vi "Window-Stage modulation program.vi"() -> ()   [LabVIEW 2020]
uses:
  Peripherals Control/XYZ Stage/Pos Modulator VIs/Typedefs/Motion Mode.ctl
  Peripherals Control/XYZ Stage/Pos Modulator VIs/Typedefs/Ops.ctl
  <vilib>/GPower/Comparison/Library/IsEven/IsEvenI32.vi
  <vilib>/GPower/Comparison/GPComparison.lvlib
panel:
  in  "Speed (um/sec)":dbl=30000.0
  in  "Z Step Size (um)":dbl=5.0
  out "stop motion local":bool
  out "error out":errorcluster
  in  "Reset":bool
  in  "stop program":bool
  in  "Stop Motion":bool
  in  "Start Motion":bool
  in  "Limit (um)":dbl=100.0
  in  "Mode":T1
  in  "Rate (Hz)":dbl=10.0
  in  "XY Step Size (um)":dbl=10.0
  # "<-- Caution !"
  # "above and below"
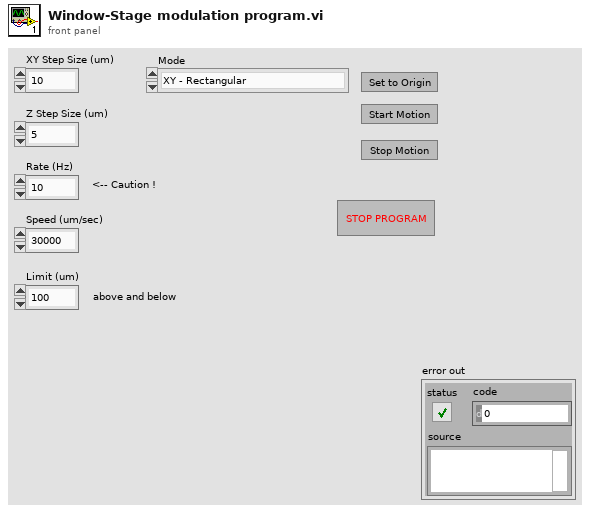
[diagram p1: front panel]
types:
  T1 = typedef "Motion Mode.ctl" = enum16{"XY - Rectangular", "XY - Random", "Z - Fixed reciprocating", "Z - Random reciprocating", "XYZ - Rectangular + Reciprocating", "XYZ Random"}
  T2 = typedef "Ops.ctl" = enum16{"Idle", "Start Motion", "Stop Motion", "Stop Program"}
  T3 = enum8{"Enabled", "Disabled", "Disabled and Grayed Out"}
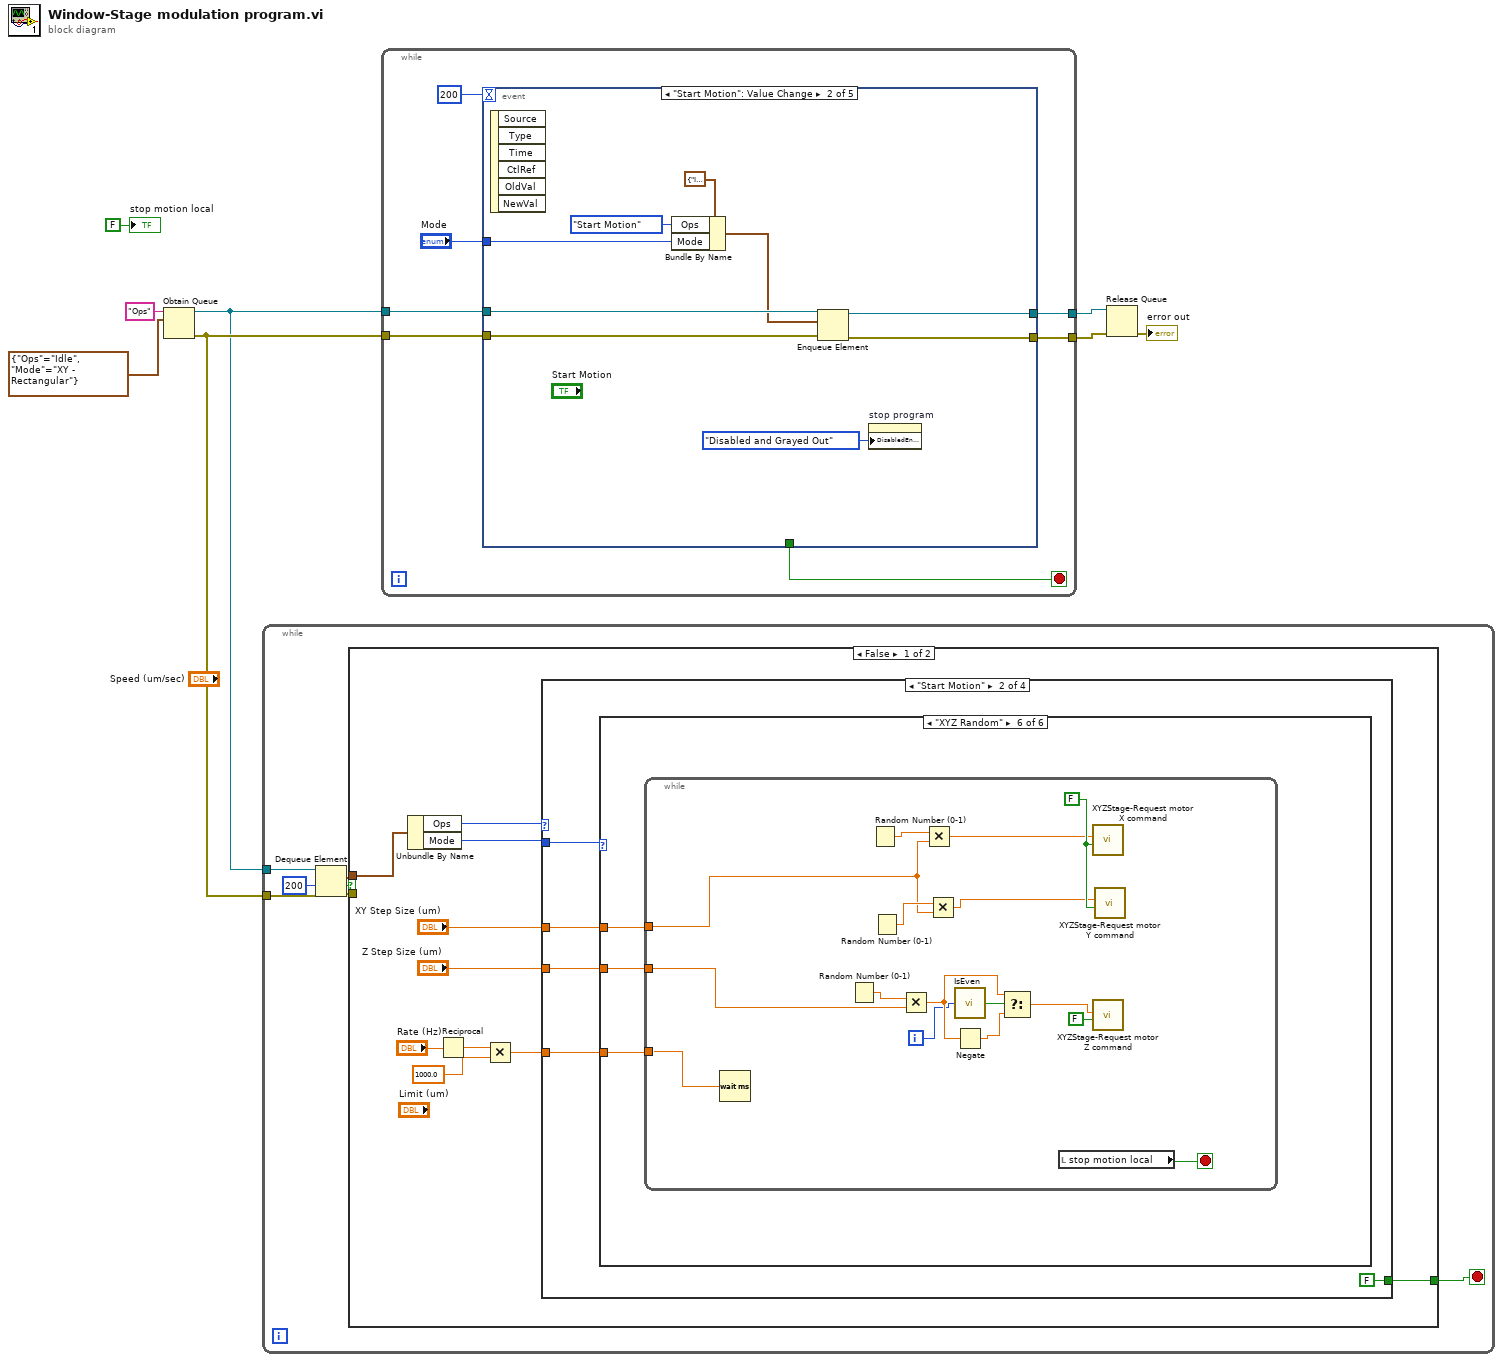
[diagram p0: block diagram]
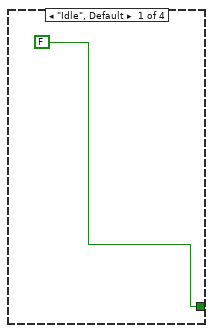
[diagram p2: hidden frame]
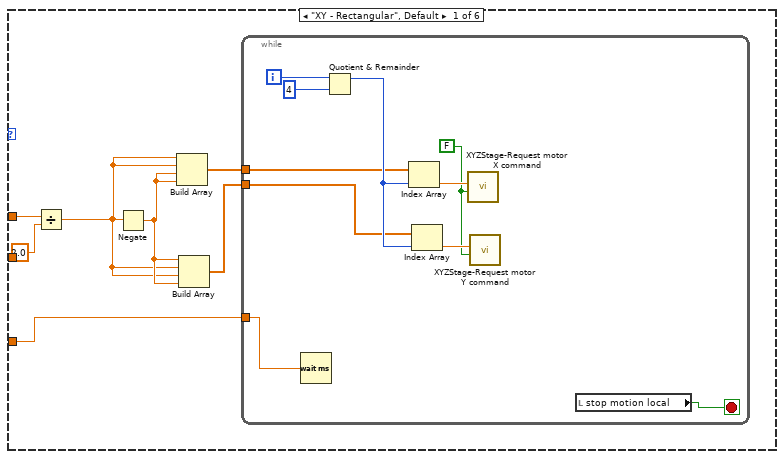
[diagram p3: hidden frame]
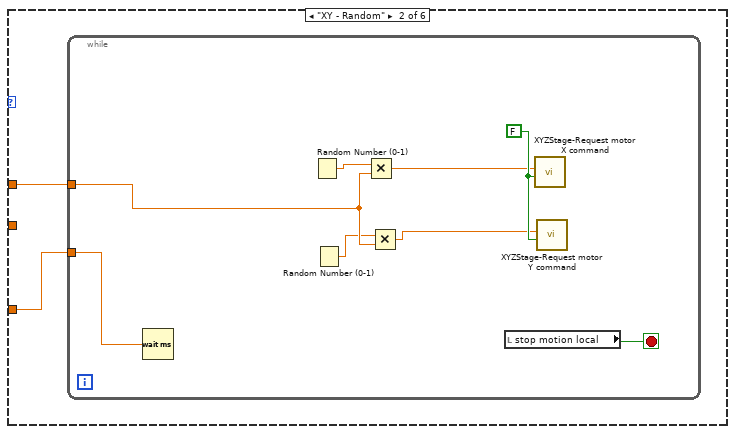
[diagram p4: hidden frame]
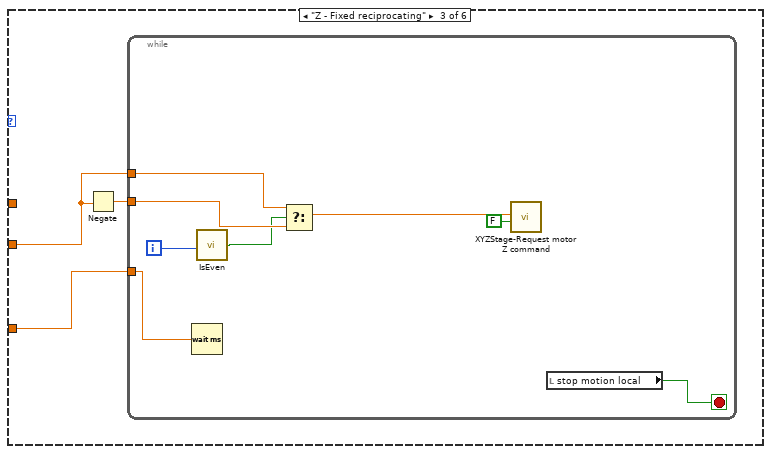
[diagram p5: hidden frame]
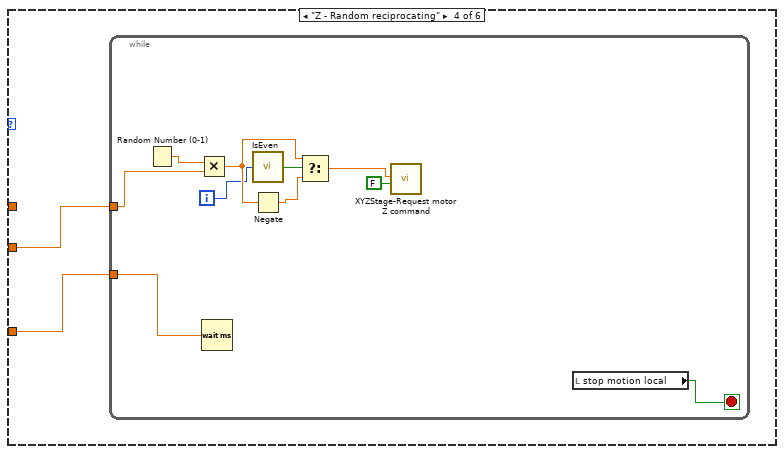
[diagram p6: hidden frame]
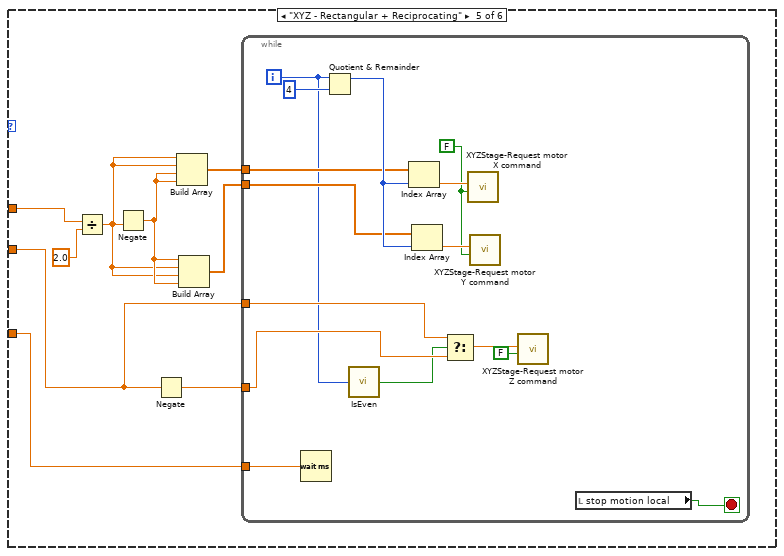
[diagram p7: hidden frame]
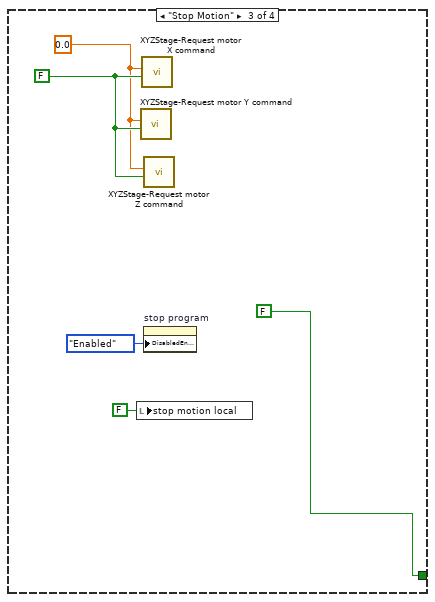
[diagram p8: hidden frame]
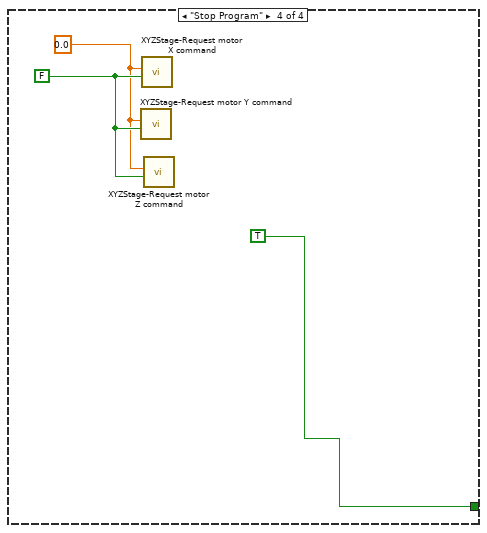
[diagram p9: hidden frame]
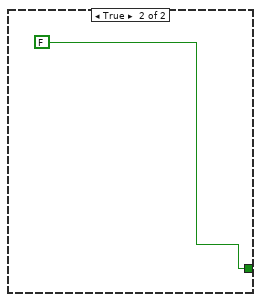
[diagram p10: hidden frame]
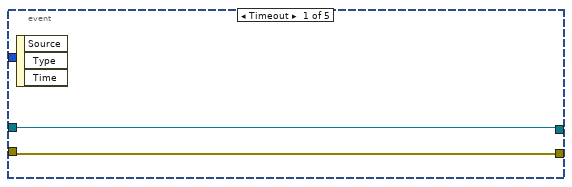
[diagram p11: hidden frame]
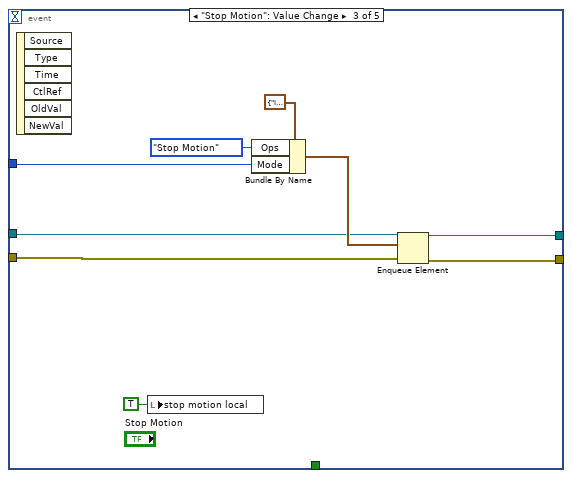
[diagram p12: hidden frame]
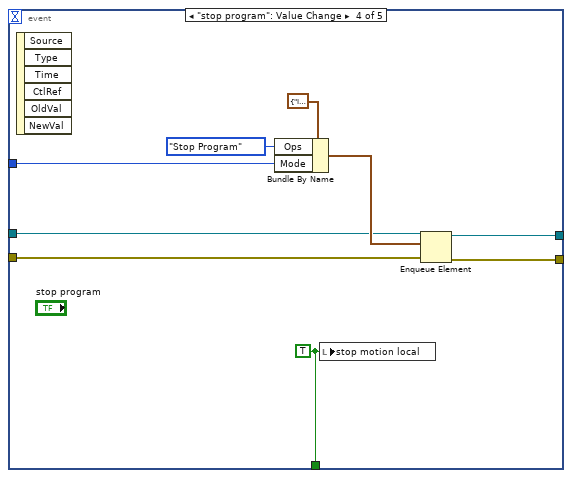
[diagram p13: hidden frame]
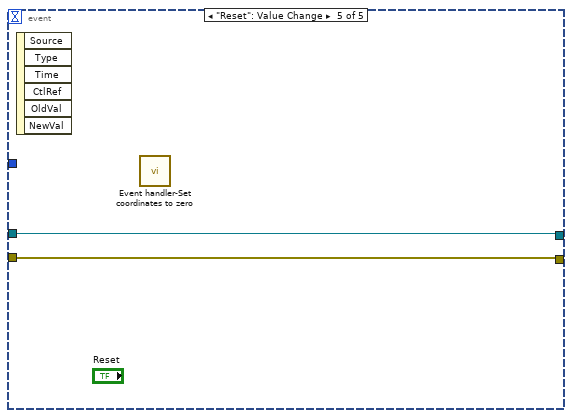
[diagram p14: hidden frame]
diagram:
  n1 = Obtain Queue(name (unnamed)="Ops", element data type=cluster{"Ops":T2, "Mode":T1} {"Ops"=enum."Idle", "Mode"=enum."XY - Rectangular"}) -> (queue out=w2:refnum<queue>, error out=w3:errorcluster)  [unwired: 3 in, 1 out]
  n2 = while {
    tunnel: w3 -> [w14]
    tunnel: w2 -> [w15]
    stop <- w9 stop-if-true
    n3 = Dequeue Element(queue=w15, timeout in ms (-1)=200, error in (no error)=w14) -> (element=w11:cluster{"Ops":T2, "Mode":T1}, timed out?=w12:bool, error out=w10:errorcluster)  [unwired: 1 out]
    n4 = case shown="False" w12 {
      tunnel: w11 -> [w25 _]
      tunnel: w10 -> [_ _]
      tunnel: [w23 FALSE] -> w9
      frame False {
        n5 = Unbundle By Name(w25) -> ("Ops"=w24:T2, "Mode"=w22:T1)
        n6 = Reciprocal(x="Rate (Hz)") -> (1/x=w19:dbl)
        n7 = Multiply(x=w19, y=1000.0) -> (x*y=w17:dbl)
        n8 = case shown="\"Start Motion\"" w24 {
          tunnel: [FALSE FALSE FALSE TRUE] -> w23
          tunnel: w22 -> [_ w30 _ _]
          tunnel: "XY Step Size (um)" -> [_ w29 _ _]
          tunnel: w17 -> [_ w28 _ _]
          tunnel: "Z Step Size (um)" -> [_ w27 _ _]
          frame "Idle", Default {
          }
          frame "Start Motion" {
            n9 = case shown="\"XYZ Random\"" w30 {
              tunnel: w29 -> [w38 w50 _ _ w83 w107]
              tunnel: w28 -> [w32 w49 w60 w71 w85 w108]
              tunnel: w27 -> [_ _ w59 w70 w82 w106]
              frame "XY - Rectangular", Default {
                n10 = Divide(x=w38, y=2.0) -> (x/y=w34:dbl)
                n11 = Negate(x=w34) -> (-x=w35:dbl)
                n12 = Build Array(w34, w34, w35, w35) -> (w36:dbl[])
                n13 = Build Array(w35, w34, w34, w35) -> (w33:dbl[])
                n14 = while {
                  tunnel: w36 -> [w40]
                  tunnel: w33 -> [w39]
                  tunnel: w32 -> [w47]
                  i -> [w46]
                  stop <- w48 stop-if-true
                  w41 = FALSE
                  n15 = Wait (ms)(milliseconds to wait=w47) -> ()  [unwired: 1 out]
                  n16 = Quotient & Remainder(x=w46, y=4) -> (x-y*floor(x/y)=w43:i32)  [unwired: 1 out]
                  n17 = Index Array(array=w40, index=w43) -> (element=w44:dbl)
                  n18 = Index Array(array=w39, index=w43) -> (element=w42:dbl)
                  n19 = call "XYZStage-Request motor X command.vi"("Wait for acknowledge?"=w41, "Motor X"=w44) -> ()  [unwired: 8 in, 2 out]
                  n20 = call "XYZStage-Request motor Y command.vi"("Wait for acknowledge?"=w41, "Motor Y"=w42) -> ()  [unwired: 8 in, 2 out]
                  n21 = local read "stop motion local"() -> (w48:bool)
                }
              }
              frame "XY - Random" {
                n22 = while {
                  tunnel: w50 -> [w55]
                  tunnel: w49 -> [w51]
                  stop <- w58 stop-if-true
                  w57 = FALSE
                  n23 = Wait (ms)(milliseconds to wait=w51) -> ()  [unwired: 1 out]
                  n24 = Random Number (0-1)() -> (number: 0 to 1=w56:dbl)
                  n25 = Random Number (0-1)() -> (number: 0 to 1=w54:dbl)
                  n26 = Multiply(x=w56, y=w55) -> (x*y=w53:dbl)
                  n27 = Multiply(x=w54, y=w55) -> (x*y=w52:dbl)
                  n28 = local read "stop motion local"() -> (w58:bool)
                  n29 = call "XYZStage-Request motor X command.vi"("Wait for acknowledge?"=w57, "Motor X"=w53) -> ()  [unwired: 8 in, 2 out]
                  n30 = call "XYZStage-Request motor Y command.vi"("Wait for acknowledge?"=w57, "Motor Y"=w52) -> ()  [unwired: 8 in, 2 out]
                }
              }
              frame "Z - Fixed reciprocating" {
                n31 = Negate(x=w59) -> (-x=w61:dbl)
                n32 = while {
                  tunnel: w59 -> [w67]
                  tunnel: w61 -> [w68]
                  tunnel: w60 -> [w64]
                  i -> [w63]
                  stop <- w69 stop-if-true
                  n33 = Wait (ms)(milliseconds to wait=w64) -> ()  [unwired: 1 out]
                  n34 = call-poly <vilib>:"IsEven.vi"("x"=w63) -> ("Even?"=w62:bool)  [unwired: 4 in]
                  n35 = Select(t=w67, s=w62, f=w68) -> (s? t:f=w66:dbl)
                  n36 = call "XYZStage-Request motor Z command.vi"("Wait for acknowledge?"=FALSE, "Motor Z"=w66) -> ()  [unwired: 7 in, 3 out]
                  n37 = local read "stop motion local"() -> (w69:bool)
                }
              }
              frame "Z - Random reciprocating" {
                n38 = while {
                  tunnel: w70 -> [w80]
                  tunnel: w71 -> [w74]
                  i -> [w72]
                  stop <- w73 stop-if-true
                  n39 = Random Number (0-1)() -> (number: 0 to 1=w81:dbl)
                  n40 = Multiply(x=w81, y=w80) -> (x*y=w78:dbl)
                  n41 = Wait (ms)(milliseconds to wait=w74) -> ()  [unwired: 1 out]
                  n42 = call-poly <vilib>:"IsEven.vi"("x"=w72) -> ("Even?"=w79:bool)  [unwired: 4 in]
                  n43 = Negate(x=w78) -> (-x=w77:dbl)
                  n44 = Select(t=w78, s=w79, f=w77) -> (s? t:f=w75:dbl)
                  n45 = call "XYZStage-Request motor Z command.vi"("Wait for acknowledge?"=FALSE, "Motor Z"=w75) -> ()  [unwired: 7 in, 3 out]
                  n46 = local read "stop motion local"() -> (w73:bool)
                }
              }
              frame "XYZ - Rectangular + Reciprocating" {
                n47 = Divide(x=w83, y=2.0) -> (x/y=w88:dbl)
                n48 = Negate(x=w88) -> (-x=w89:dbl)
                n49 = Negate(x=w82) -> (-x=w84:dbl)
                n50 = Build Array(w88, w88, w89, w89) -> (w90:dbl[])
                n51 = Build Array(w89, w88, w88, w89) -> (w87:dbl[])
                n52 = while {
                  tunnel: w90 -> [w98]
                  tunnel: w87 -> [w97]
                  tunnel: w85 -> [w104]
                  tunnel: w84 -> [w93]
                  tunnel: w82 -> [w94]
                  i -> [w92]
                  stop <- w105 stop-if-true
                  w99 = FALSE
                  n53 = Wait (ms)(milliseconds to wait=w104) -> ()  [unwired: 1 out]
                  n54 = Quotient & Remainder(x=w92, y=4) -> (x-y*floor(x/y)=w101:i32)  [unwired: 1 out]
                  n55 = call-poly <vilib>:"IsEven.vi"("x"=w92) -> ("Even?"=w91:bool)  [unwired: 4 in]
                  n56 = Index Array(array=w98, index=w101) -> (element=w102:dbl)
                  n57 = Index Array(array=w97, index=w101) -> (element=w100:dbl)
                  n58 = Select(t=w94, s=w91, f=w93) -> (s? t:f=w96:dbl)
                  n59 = call "XYZStage-Request motor X command.vi"("Wait for acknowledge?"=w99, "Motor X"=w102) -> ()  [unwired: 8 in, 2 out]
                  n60 = call "XYZStage-Request motor Y command.vi"("Wait for acknowledge?"=w99, "Motor Y"=w100) -> ()  [unwired: 8 in, 2 out]
                  n61 = call "XYZStage-Request motor Z command.vi"("Wait for acknowledge?"=FALSE, "Motor Z"=w96) -> ()  [unwired: 7 in, 3 out]
                  n62 = local read "stop motion local"() -> (w105:bool)
                }
              }
              frame "XYZ Random" {
                n63 = while {
                  tunnel: w107 -> [w111]
                  tunnel: w108 -> [w118]
                  tunnel: w106 -> [w110]
                  i -> [w109]
                  stop <- w124 stop-if-true
                  w123 = FALSE
                  n64 = Wait (ms)(milliseconds to wait=w118) -> ()  [unwired: 1 out]
                  n65 = Random Number (0-1)() -> (number: 0 to 1=w117:dbl)
                  n66 = Random Number (0-1)() -> (number: 0 to 1=w122:dbl)
                  n67 = Random Number (0-1)() -> (number: 0 to 1=w121:dbl)
                  n68 = Multiply(x=w117, y=w110) -> (x*y=w115:dbl)
                  n69 = Multiply(x=w122, y=w111) -> (x*y=w120:dbl)
                  n70 = Multiply(x=w121, y=w111) -> (x*y=w119:dbl)
                  n71 = call-poly <vilib>:"IsEven.vi"("x"=w109) -> ("Even?"=w116:bool)  [unwired: 4 in]
                  n72 = Negate(x=w115) -> (-x=w114:dbl)
                  n73 = Select(t=w115, s=w116, f=w114) -> (s? t:f=w112:dbl)
                  n74 = local read "stop motion local"() -> (w124:bool)
                  n75 = call "XYZStage-Request motor X command.vi"("Wait for acknowledge?"=w123, "Motor X"=w120) -> ()  [unwired: 8 in, 2 out]
                  n76 = call "XYZStage-Request motor Z command.vi"("Wait for acknowledge?"=FALSE, "Motor Z"=w112) -> ()  [unwired: 7 in, 3 out]
                  n77 = call "XYZStage-Request motor Y command.vi"("Wait for acknowledge?"=w123, "Motor Y"=w119) -> ()  [unwired: 8 in, 2 out]
                }
              }
            }
          }
          frame "Stop Motion" {
            w127 = sgl 0.0 ("Motor X")
            w128 = FALSE ("Wait for acknowledge?")
            n78 = local write "stop motion local"(FALSE ("stop motion local")) -> ()
            n79 = call "XYZStage-Request motor Y command.vi"("Wait for acknowledge?"=w128, "Motor Y"=w127) -> ()  [unwired: 8 in, 2 out]
            n80 = call "XYZStage-Request motor X command.vi"("Wait for acknowledge?"=w128, "Motor X"=w127) -> ()  [unwired: 8 in, 2 out]
            n81 = call "XYZStage-Request motor Z command.vi"("Wait for acknowledge?"=w128, "Motor Z"=w127) -> ()  [unwired: 7 in, 3 out]
            n82 = property on="stop program" class="Bool"("DisabledEnum"=T3."Enabled" ("Disabled")) -> ()  [unwired: 2 in, 2 out]
          }
          frame "Stop Program" {
            w130 = sgl 0.0 ("Motor X")
            w131 = FALSE ("Wait for acknowledge?")
            n83 = call "XYZStage-Request motor Y command.vi"("Wait for acknowledge?"=w131, "Motor Y"=w130) -> ()  [unwired: 8 in, 2 out]
            n84 = call "XYZStage-Request motor X command.vi"("Wait for acknowledge?"=w131, "Motor X"=w130) -> ()  [unwired: 8 in, 2 out]
            n85 = call "XYZStage-Request motor Z command.vi"("Wait for acknowledge?"=w131, "Motor Z"=w130) -> ()  [unwired: 7 in, 3 out]
          }
        }
      }
      frame True {
      }
    }
  }
  n86 = while {
    tunnel: w2 -> [w139]
    tunnel: w3 -> [w138]
    tunnel: [w136] -> w5
    tunnel: [w135] -> w6
    stop <- w134 stop-if-true
    n87 = event shown="[1] \"Start Motion\": Value Change" {
      selector: _ -> [_ _ _ _ _]
      dyn-events: _ -> [_ _ _ _ _]
      timeout: 200 -> [_ _ _ _ _]
      tunnel: w139 -> [w142 w151 w156 w166 w171]
      tunnel: w138 -> [w141 w150 w157 w165 w170]
      tunnel: "Mode" -> [_ w146 w153 w162 _]
      tunnel: [w142 w145 w155 w164 w171] -> w136
      tunnel: [w141 w144 w154 w163 w170] -> w135
      tunnel: [_ _ _ w161 _] -> w134
      event Timeout {
        n88 = event-data() -> ()  [unwired: 1 in, 3 out]
      }
      event "Start Motion": Value Change {
        n89 = event-data() -> ()  [unwired: 1 in, 6 out]
        n90 = Bundle By Name(cluster=cluster{"Ops":T2, "Mode":T1} {"Ops"=enum."Idle", "Mode"=enum."XY - Rectangular"}, "Ops"=Ops."Start Motion", "Mode"=w146) -> (w149:cluster{"Ops":T2, "Mode":T1})
        n91 = Enqueue Element(queue=w151, element=w149, error in (no error)=w150) -> (queue out=w145:refnum<queue>, error out=w144:errorcluster)  [unwired: 1 in, 1 out]
        n92 = property on="stop program" class="Bool"("DisabledEnum"=T3."Disabled and Grayed Out" ("Disabled")) -> ()  [unwired: 2 in, 2 out]
      }
      event "Stop Motion": Value Change {
        n93 = event-data() -> ()  [unwired: 1 in, 6 out]
        n94 = local write "stop motion local"(TRUE ("stop motion local")) -> ()
        n95 = Bundle By Name(cluster=cluster{"Ops":T2, "Mode":T1} {"Ops"=enum."Idle", "Mode"=enum."XY - Rectangular"}, "Ops"=Ops."Stop Motion", "Mode"=w153) -> (w160:cluster{"Ops":T2, "Mode":T1})
        n96 = Enqueue Element(queue=w156, element=w160, error in (no error)=w157) -> (queue out=w155:refnum<queue>, error out=w154:errorcluster)  [unwired: 1 in, 1 out]
      }
      event "stop program": Value Change {
        w161 = TRUE ("stop motion local")
        n97 = event-data() -> ()  [unwired: 1 in, 6 out]
        n98 = Bundle By Name(cluster=cluster{"Ops":T2, "Mode":T1} {"Ops"=enum."Idle", "Mode"=enum."XY - Rectangular"}, "Ops"=Ops."Stop Program", "Mode"=w162) -> (w169:cluster{"Ops":T2, "Mode":T1})
        n99 = local write "stop motion local"(w161) -> ()
        n100 = Enqueue Element(queue=w166, element=w169, error in (no error)=w165) -> (queue out=w164:refnum<queue>, error out=w163:errorcluster)  [unwired: 1 in, 1 out]
      }
      event "Reset": Value Change {
        n101 = event-data() -> ()  [unwired: 1 in, 6 out]
        n102 = call "Event handler-Set coordinates to zero.vi"() -> ()  [unwired: 12 in]
      }
    }
  }
  n103 = Release Queue(queue=w5, error in (no error)=w6) -> (error out=→"error out":errorcluster)  [unwired: 1 in, 2 out]
  "stop motion local" <- FALSE ("stop motion local")
